vi "PH_ForceSensor.Calculate Forces.vi"(0 "VI in":refnum<vi>, 5 "error in":errorcluster) -> (14 "VI out":refnum<vi>, 19 "error out":errorcluster)   [LabVIEW 2014, in "PH_ForceSensor.lvlib"]
uses:
  PH_ForceSensor.lvlib
  PH_Common/PH_Common.lvlib
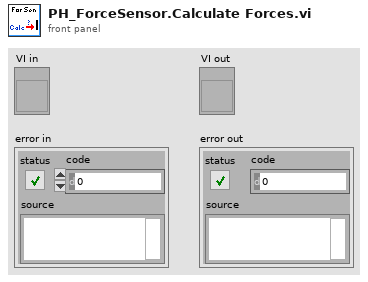
[diagram p1: front panel]
types:
  T1 = typedef "PH_ForceSensor.lvlib/PH_ForceSensor.i attribute.ctl" = cluster{"GUI Refs":T2, "Rawvalues":T3, "Offsets [µV]":T3, "Scalings [mV/V]":T3, "Forces [N]":T3, "Supply Voltage [V]":dbl, "Full Force [N]":dbl, "Ranges [N]":cluster{"Low Energy":cluster{"Upper Limit":dbl, "Lower Limit":dbl}, "High Energy":cluster{"Upper Limit":dbl, "Lower Limit":dbl}}}
  T2 = typedef "PH_ForceSensor.lvlib/PH_ForceSensor.GUI Refs.ctl" = cluster{"Delete":refnum<vi>, "Rawvalues":refnum<vi>, "Offsets [µV]":refnum<vi>, "Sensor Values [µV]":refnum<vi>, "Scalings [mV/V]":refnum<vi>, "Supply Voltage [V]":refnum<vi>, "Full Force [N]":refnum<vi>, "Forces [N]":refnum<vi>, "Graph Differential Forces":refnum<vi>, "Graph Absolute Forces":refnum<vi>, "Ranges [N]":refnum<vi>}
  T3 = typedef "PH_ForceSensor.lvlib/PH_ForceSensor.Dataset.ctl" = cluster{"top front":dbl, "top back":dbl, "bottom front":dbl, "bottom back":dbl}
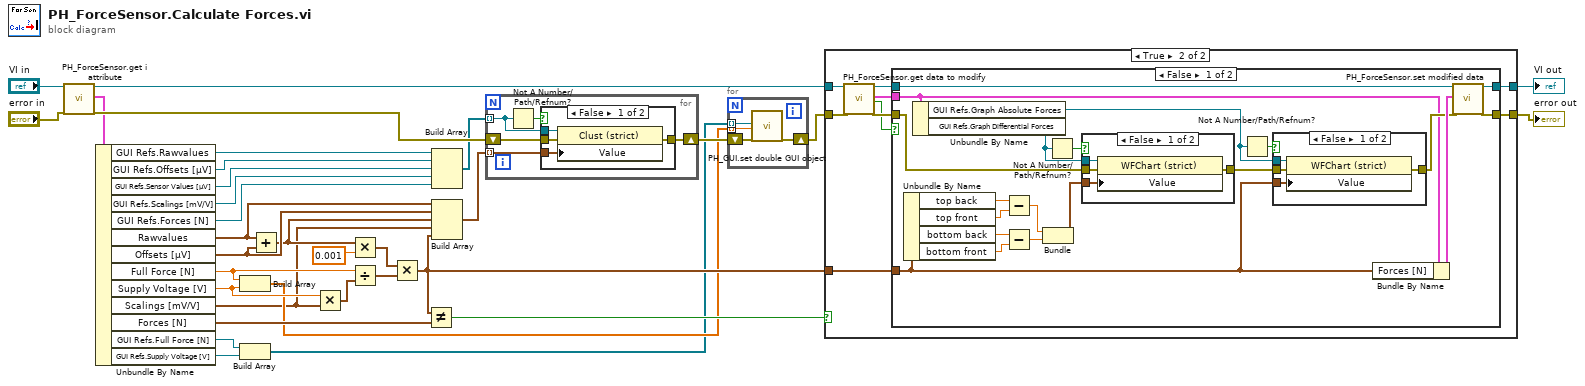
[diagram p0: block diagram]
diagram:
  n1 = call "PH_ForceSensor.get i attribute.vi"("i ref in"="VI in", "error in (no error)"="error in") -> ("i ref out"=w33:refnum<vi>, "i attribute"=w29:T1, "error out"=w31:errorcluster)  [unwired: 15 in]
  n2 = Unbundle By Name(w29) -> ("GUI Refs.Rawvalues"=w28:refnum<vi>, "GUI Refs.Offsets [µV]"=w27:refnum<vi>, "GUI Refs.Sensor Values [µV]"=w3:refnum<vi>, "GUI Refs.Scalings [mV/V]"=w19:refnum<vi>, "GUI Refs.Forces [N]"=w18:refnum<vi>, "Rawvalues"=w25:T3, "Offsets [µV]"=w4:T3, "Full Force [N]"=w9:dbl, "Supply Voltage [V]"=w10:dbl, "Scalings [mV/V]"=w1:T3, "Forces [N]"=w13:T3, "GUI Refs.Full Force [N]"=w6:refnum<vi>, "GUI Refs.Supply Voltage [V]"=w7:refnum<vi>)
  n3 = Build Array(w9, w10) -> (w8:dbl[])
  n4 = Build Array(w6, w7) -> (w5:refnum<vi>[])
  n5 = Add(x=w25, y=w4) -> (x+y=w2:T3)
  n6 = Multiply(x=w10, y=w1) -> (x*y=w21:T3)
  n7 = Multiply(x=w2, y=0.001) -> (x*y=w22:T3)
  n8 = Divide(x=w9, y=w21) -> (x/y=w20:T3)
  n9 = Multiply(x=w22, y=w20) -> (x*y=w14:T3)
  n10 = Not Equal?(x=w14, y=w13) -> (x != y?=w12:bool)
  n11 = Build Array(w28, w27, w3, w19, w18) -> (w26:refnum<vi>[])
  n12 = Build Array(w25, w4, w2, w1, w14) -> (w24:T3[])
  n13 = for {
    shift-right: [w37] -> w16
    shift-left: w31 -> [w38]
    tunnel: w26 -> [w35] mode=indexing
    tunnel: w24 -> [w34] mode=indexing
    n14 = Not A Number/Path/Refnum?(number/path/refnum=w35) -> (NaN/Path/Refnum?=w36:bool)
    n15 = case shown="False" w36 {
      tunnel: w38 -> [w42 w43]
      tunnel: [w41 w43] -> w37
      tunnel: w35 -> [w40 _]
      tunnel: w34 -> [w39 _]
      frame False {
        n16 = property class="Clust (strict)"(reference=w40, error in=w42, "Value"=w39) -> (error out=w41:errorcluster)  [unwired: 1 out]
      }
      frame True {
      }
    }
  }
  n17 = for {
    tunnel: w8 -> [w45] mode=indexing
    shift-right: [w46] -> w11
    shift-left: w16 -> [w47]
    tunnel: w5 -> [w44] mode=indexing
    n18 = call "PH_GUI.set double GUI object.vi"("GUI object Ref"=w44, "value"=w45, "error in (no error)"=w47) -> ("error out"=w46:errorcluster)  [unwired: 16 in]
  }
  n19 = case shown="True" w12 {
    tunnel: w33 -> [w49 w58]
    tunnel: [w49 w56] -> w17
    tunnel: w11 -> [w48 w53]
    tunnel: [w48 w52] -> w15
    tunnel: w14 -> [_ w50]
    frame False {
    }
    frame True {
      n20 = call "PH_ForceSensor.get data to modify.vi"("i ref in"=w58, "error in (no error)"=w53) -> ("i ref out"=w57:refnum<vi>, "i attribute"=w54:T1, "timed out"=w51:bool, "error out"=w55:errorcluster)  [unwired: 14 in]
      n21 = case shown="False" w51 {
        tunnel: w57 -> [w78 w90]
        tunnel: [w77 w90] -> w56
        tunnel: w55 -> [w70 w89]
        tunnel: w54 -> [w67 _]
        tunnel: [w76 w89] -> w52
        tunnel: w50 -> [w63 _]
        frame False {
          n22 = Unbundle By Name(w63) -> ("top back"=w74:dbl, "top front"=w73:dbl, "bottom back"=w72:dbl, "bottom front"=w71:dbl)
          n23 = Unbundle By Name(w67) -> ("GUI Refs.Graph Absolute Forces"=w60:refnum<vi>, "GUI Refs.Graph Differential Forces"=w62:refnum<vi>)
          n24 = Subtract(x=w74, y=w73) -> (x-y=w66:dbl)
          n25 = Subtract(x=w72, y=w71) -> (x-y=w65:dbl)
          n26 = Bundle(w66, w65) -> (w64:cluster{dbl, dbl})  [unwired: 1 in]
          n27 = Not A Number/Path/Refnum?(number/path/refnum=w62) -> (NaN/Path/Refnum?=w61:bool)
          n28 = case shown="False" w61 {
            tunnel: w70 -> [w87 w88]
            tunnel: [w86 w88] -> w69
            tunnel: w62 -> [w85 _]
            tunnel: w64 -> [w84 _]
            frame False {
              n29 = property class="WFChart (strict)"(reference=w85, error in=w87, "Value"=w84) -> (error out=w86:errorcluster)  [unwired: 1 out]
            }
            frame True {
            }
          }
          n30 = Not A Number/Path/Refnum?(number/path/refnum=w60) -> (NaN/Path/Refnum?=w59:bool)
          n31 = case shown="False" w59 {
            tunnel: w69 -> [w82 w83]
            tunnel: [w81 w83] -> w68
            tunnel: w60 -> [w80 _]
            tunnel: w63 -> [w79 _]
            frame False {
              n32 = property class="WFChart (strict)"(reference=w80, error in=w82, "Value"=w79) -> (error out=w81:errorcluster)  [unwired: 1 out]
            }
            frame True {
            }
          }
          n33 = Bundle By Name(cluster=w67, "Forces [N]"=w63) -> (w75:T1)
          n34 = call "PH_ForceSensor.set modified data.vi"("i ref in"=w78, "i attribute"=w75, "error in (no error)"=w68) -> ("i ref out"=w77:refnum<vi>, "error out"=w76:errorcluster)  [unwired: 15 in]
        }
        frame True {
        }
      }
    }
  }
  "VI out" <- w17
  "error out" <- w15
